vi "Coord window-Edit cell handler.vi"   [LabVIEW 2017]
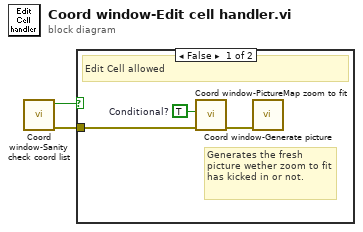
[diagram p0: block diagram]
diagram:
  n1 = call "Coord window-Sanity check coord list.vi"() -> ("error out"=w1:errorcluster, "Discard"=w2:bool)  [unwired: 10 in]
  n2 = case shown="False" w2 {
    tunnel: w1 -> [w4 _]
    frame False {
      w5 = TRUE  # Conditional?
      # "Generates the fresh picture wether zoom to fit has kicked in or not."
      # "Edit Cell allowed"
      n3 = call "Coord window-PictureMap zoom to fit.vi"("error in"=w4, "Conditional?"=w5) -> ("error out"=w3:errorcluster)  [unwired: 9 in]
      n4 = call "Coord window-Generate picture.vi"("error in (no error)"=w3) -> ()  [unwired: 10 in, 1 out]
    }
    frame True {
      # "Discarded"
    }
  }
